vi "Sensor_Simulator.vi"(2 "Loop Rate (ms)":i64=10, 3 "initialize":bool, 5 "Velocity":dbl(knob)=1.0013024669594606 scale=0.0..10.0, 7 "Input":dbl format="%0.2f") -> (1 "Position":dbl format="%0.2f")   [LabVIEW 2016]
uses:
  <vilib>/ptbypt/NI_PtbyPt.lvlib
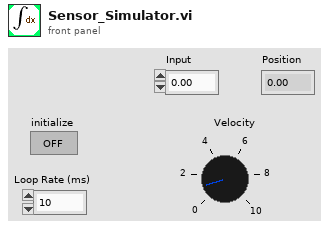
[diagram p1: front panel]
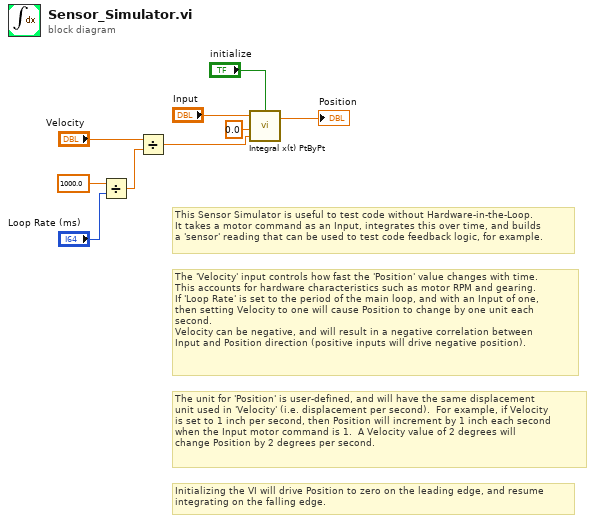
[diagram p0: block diagram]
diagram:
  # "Initializing the VI will drive Position to zero on the leading edge, and resume\nintegrating on the falling edge."
  # "The unit for 'Position' is user-defined, and will have the same displacement\nunit used in 'Velocity' (i.e. displacement per second).  For example, if Velocity\nis set to 1 inch per second, then Position will increment by 1 inch each second\nwhen the Input motor command is 1.  A Velocity value of 2 degrees will \nchange Position by 2 degrees per second."
  # "The 'Velocity' input controls how fast the 'Position' value changes with time.\nThis accounts for hardware characteristics such as motor RPM and gearing.\nIf 'Loop Rate' is set to the period of the main loop, and with an Input of one, \nthen setting Velocity to one will cause Position to change by one unit each \nsecond.\nVelocity can be negative, and will result in a negative correlation between\nInput and Position direction (positive inputs will drive negative position)."
  # "This Sensor Simulator is useful to test code without Hardware-in-the-Loop.\nIt takes a motor command as an Input, integrates this over time, and builds\na 'sensor' reading that can be used to test code feedback logic, for example."
  n1 = Divide(x=1000.0, y="Loop Rate (ms)") -> (x/y=w4:dbl)
  n2 = Divide(x="Velocity", y=w4) -> (x/y=w5:dbl)
  n3 = call <vilib>:"Integral x(t) PtByPt.vi"("initialize"="initialize", "dt"=w5, "initial condition"=0.0, "x"="Input") -> ("integral x(t)"=→"Position":dbl)  [unwired: 1 out]
